vi "Query Client for Token.vi"(8 "error in (no error)":errorcluster, 10 "Request URI":string, 11 "OAuthClient in":refnum<class "OAuthClient.lvclass">) -> (0 "error out":errorcluster, 1 "Body":string, 2 "Header":string, 3 "OAuthClient out":refnum<class "OAuthClient.lvclass">)   [LabVIEW 2017, in "OAuthClient.lvclass"]
uses:
  OAuthClient.lvclass
  OAuthClient.lvclass/OAuthClient.ctl
  <vilib>/httpClient/POSTBuffer.vi
  <vilib>/httpClient/LabVIEWHTTPClient.lvlib
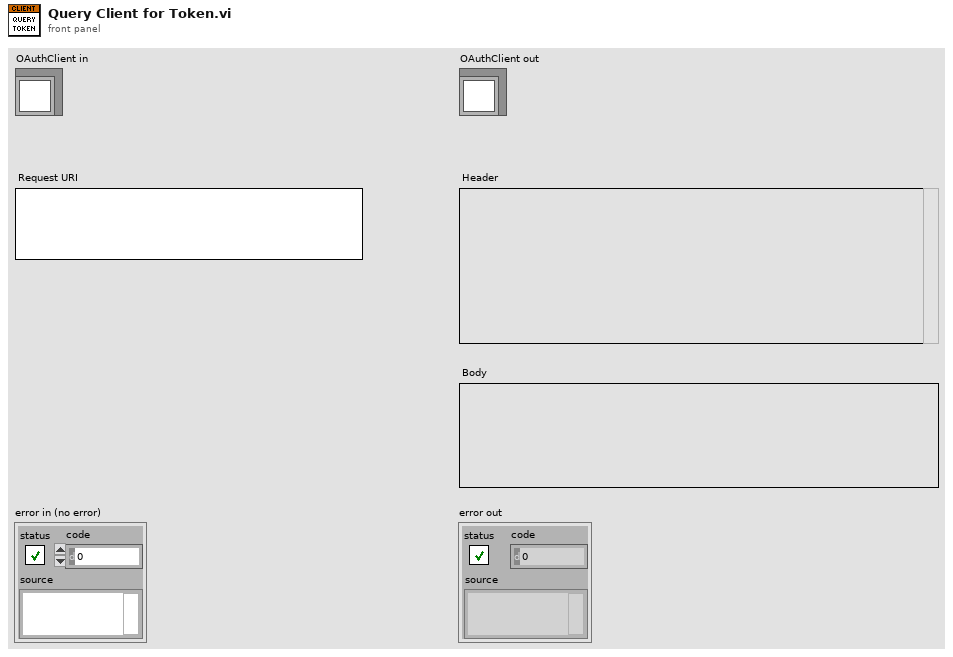
[diagram p1: front panel]
types:
  T1 = typedef "LabVIEWHTTPClient.lvlib/ClientHandle.ctl" = refnum<k1>
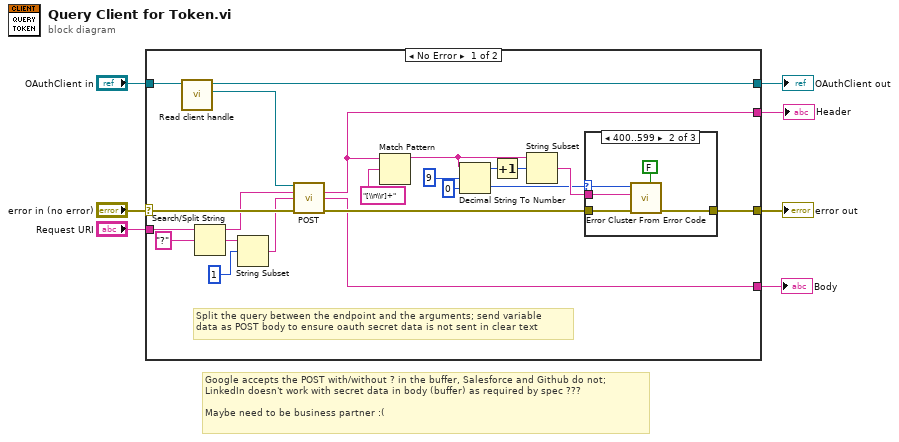
[diagram p0: block diagram]
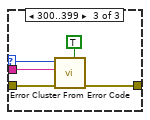
[diagram p3: hidden frame]
diagram:
  # "Google accepts the POST with/without ? in the buffer, Salesforce and Github do not;\nLinkedIn doesn't work with secret data in body (buffer) as required by spec ???\n\nMaybe need to be business partner :("
  n1 = case shown="No Error" "error in (no error)" {
    selector: "error in (no error)" -> [w15 w42]
    tunnel: [w19 w42] -> w6
    tunnel: [w28 w41] -> w4
    tunnel: "OAuthClient in" -> [w29 w41]
    tunnel: "Request URI" -> [w11 _]
    tunnel: [w18 _] -> w2
    tunnel: [w16 _] -> w1
    frame No Error {
      # "Split the query between the endpoint and the arguments; send variable \ndata as POST body to ensure oauth secret data is not sent in clear text"
      n2 = call "Read client handle.vi"("OAuthClient in"=w29) -> ("Client Handle"=w14:T1, "OAuthClient out"=w28:refnum<class "OAuthClient.lvclass">)  [unwired: 8 in, 1 out]
      n3 = Search/Split String(string=w11, search string/char (-)="?") -> (substring before match=w10:string, match + rest of string=w9:string)  [unwired: 1 in, 1 out]
      n4 = String Subset(string=w9, offset (0)=1) -> (substring=w8:string)  [unwired: 1 in]
      n5 = call-poly <vilib>:"POST.vi"("client handle"=w14, "url"=w10, "buffer"=w8, "error in (no error)"=w15) -> ("headers"=w16:string, "body"=w18:string, "error out"=w20:errorcluster)  [unwired: 8 in, 1 out]
      n6 = Match Pattern(string=w16, regular expression="[\\n\\r]+") -> (before substring=w26:string)  [unwired: 1 in, 3 out]
      n7 = Decimal String To Number(string=w26, offset=u32 9 ("initial scan location"), default (0L)=0 ("default value 1")) -> (offset past number=w24:i32, number=w23:i32)
      n8 = Increment(x=w24) -> (x+1=w27:i32)
      n9 = String Subset(string=w26, offset (0)=w27) -> (substring=w25:string)  [unwired: 1 in]
      n10 = case shown="400..599" w23 {
        selector: w23 -> [_ w33 w38]
        tunnel: w20 -> [w30 w35 w40]
        tunnel: [w30 w34 w39] -> w19
        tunnel: w25 -> [_ w32 w37]
        frame Default {
        }
        frame 400..599 {
          n11 = call <vilib>:"Error Cluster From Error Code.vi"("is warning? (False)"=FALSE, "error in (no error)"=w35, "error message (\"\")"=w32, "error code (0)"=w33) -> ("error out"=w34:errorcluster)  [unwired: 5 in]
        }
        frame 300..399 {
          n12 = call <vilib>:"Error Cluster From Error Code.vi"("is warning? (False)"=TRUE, "error in (no error)"=w40, "error message (\"\")"=w37, "error code (0)"=w38) -> ("error out"=w39:errorcluster)  [unwired: 5 in]
        }
      }
    }
    frame Error {
    }
  }
  "error out" <- w6
  "OAuthClient out" <- w4
  "Body" <- w2
  "Header" <- w1
